vi "read_text_file.vi"(2 "error in (no error)":errorcluster, 3 "file_path":path=path "C:/luminartech/ManufacturingTools/TS_Automation/Programs/Labview/bring_up/hbEnable/hbEnable_resp.txt") -> (0 "error out":errorcluster, 1 "text":string)   [LabVIEW 2018]
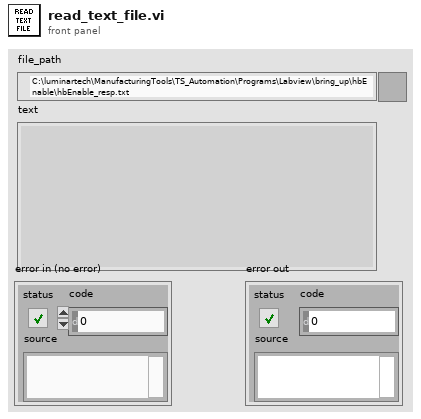
[diagram p1: front panel]
types:
  T1 = enum16{"open", "replace", "create", "open or create", "replace or create", "replace or create with confirmation"}
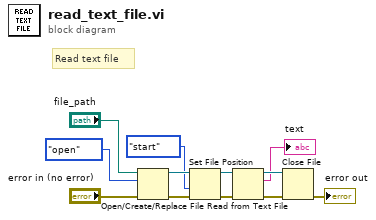
[diagram p0: block diagram]
diagram:
  # "Read text file"
  n1 = Open/Create/Replace File(file path (use dialog)="file_path", error in="error in (no error)", operation (0:open)=T1."open") -> (refnum out=w11:refnum<file>, error out=w8:errorcluster)  [unwired: 3 in, 1 out]
  n2 = Set File Position(refnum=w11, from (0:start)=enum16{"start", "end", "current"}."start", error in=w8) -> (refnum out=w10:refnum<file>, error out=w7:errorcluster)  [unwired: 1 in]
  n3 = Read from Text File(file (use dialog)=w10, error in=w7) -> (refnum out=w9:refnum<file>, text=→"text":string, error out=w6:errorcluster)  [unwired: 2 in, 1 out]
  n4 = Close File(refnum=w9, error in=w6) -> (error out=→"error out":errorcluster)  [unwired: 1 out]
